vi "Audio Device Capture Example (G-Audio).vi"() -> ()   [LabVIEW 2020]
doc: "Simple example of audio device capture, saving the acquired data to a WAV file."
uses:
  Controls/Audio Device Config.ctl
  Controls/Audio Device Format.ctl
  Controls/Audio Device Info.ctl
  Controls/Audio Device Type.ctl
  Controls/Audio File Info.ctl
  Controls/WAV Codec Specific Info.ctl
  Controls/WAV Container Format.ctl
  Controls/WAV Data Format.ctl
  d37775a1-27ef-4781-ba3e-b38a0bb78134.vi
  7b5afa26-ffc7-4768-ab84-ffe08a27723a.vi
  Private/Result To Error.vi
  d37775a1-27ef-4781-ba3e-b38a0bb78134.vi/6b901882-6109-4f44-aca5-48e1525e5248.vi
  d37775a1-27ef-4781-ba3e-b38a0bb78134.vi/06c0137a-63d3-4e30-982f-115d83a1188c.vi
  Private/Get Configured Audio Device Info.vi
  7b5afa26-ffc7-4768-ab84-ffe08a27723a.vi/fba40667-3e21-44fa-934c-95909d78721c.vi
  d37775a1-27ef-4781-ba3e-b38a0bb78134.vi/6b901882-6109-4f44-aca5-48e1525e5248.vi/a9d2058a-38f9-4c88-a1a9-9bf864ebbde5.vi
  d37775a1-27ef-4781-ba3e-b38a0bb78134.vi/06c0137a-63d3-4e30-982f-115d83a1188c.vi/4b7b629c-2e91-4160-9820-a26af8f6e677.vi
  d37775a1-27ef-4781-ba3e-b38a0bb78134.vi/06c0137a-63d3-4e30-982f-115d83a1188c.vi/e7c4a249-ce38-42b4-8985-5fdb76b4ebfc.vi
  7b5afa26-ffc7-4768-ab84-ffe08a27723a.vi/fba40667-3e21-44fa-934c-95909d78721c.vi/4b7b629c-2e91-4160-9820-a26af8f6e677.vi
  7b5afa26-ffc7-4768-ab84-ffe08a27723a.vi/fba40667-3e21-44fa-934c-95909d78721c.vi/e7c4a249-ce38-42b4-8985-5fdb76b4ebfc.vi
  Audio Files/Polymorphic VIs/Open Audio File Write (WAV).vi
  <vilib>/Utility/Data Type/Get Numeric Information.vi
  <vilib>/Utility/error.llb/Error Cluster From Error Code.vi
  G-Audio.lvlib
panel:
  out "error out":errorcluster
  in  "Stop":bool
  out "Waveform":waveform(i16)[](graph)
  # "Instructions:\n1. Run the VI.\n2. Choose a WAV file location to save the captured audio data to.\n3. The VI will begin audio capture and display the data in the waveform graph.\n4. Press Stop to finish audio capture, and save the WAV fle.\n5. Listen to the recorded WAV with Audio Device Playback Example (G-Audio).vi."
  # "G"
  # "-Audio"
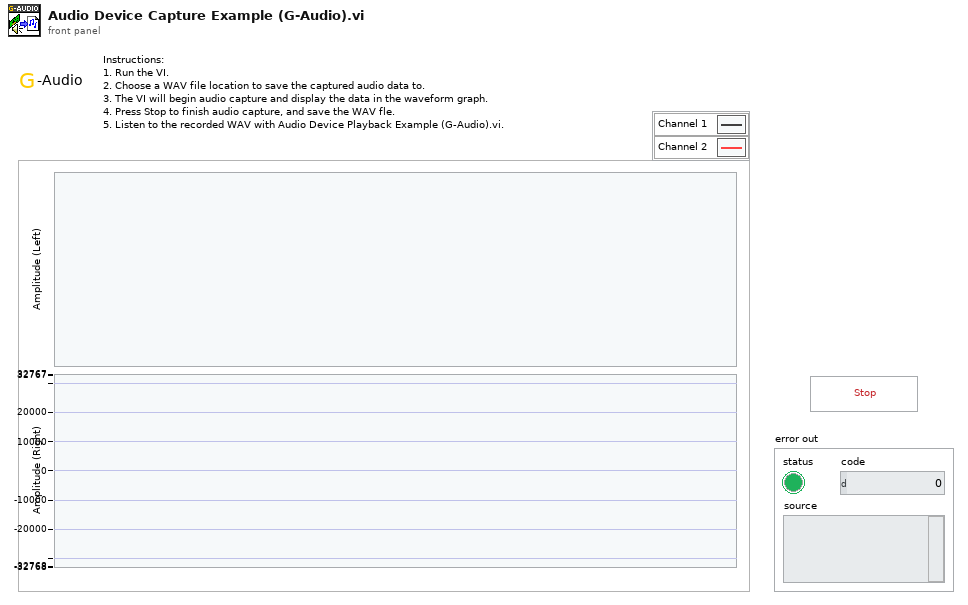
[diagram p1: front panel]
types:
  T1 = typedef "G-Audio.lvlib/WAV Codec Specific Info.ctl" = cluster{"Container Format":T2, "Data Format":T3}
  T2 = typedef "G-Audio.lvlib/WAV Container Format.ctl" = enum32{"RIFF", "Wave64"}
  T3 = typedef "G-Audio.lvlib/WAV Data Format.ctl" = u32
  T4 = typedef "G-Audio.lvlib/Audio File Info.ctl" = cluster{"Sample Rate (Hz)":u32, "Channels":u32, "Bit Depth":u32}
  T5 = typedef "G-Audio.lvlib/Audio Device Info.ctl" = cluster{"Name":string, "ID":u8[], "Device Type":T6}
  T6 = typedef "G-Audio.lvlib/Audio Device Type.ctl" = enum16{"(None)", "Playback", "Capture", "Duplex", "Loopback"}
  T7 = typedef "G-Audio.lvlib/Audio Device Config.ctl" = cluster{"Sample Rate (Hz)":u32, "Channels":u32, "Format":T8, "Exclusive Mode":bool}
  T8 = typedef "G-Audio.lvlib/Audio Device Format.ctl" = enum16{"Native", "U8", "I16", "I32", "SGL"}
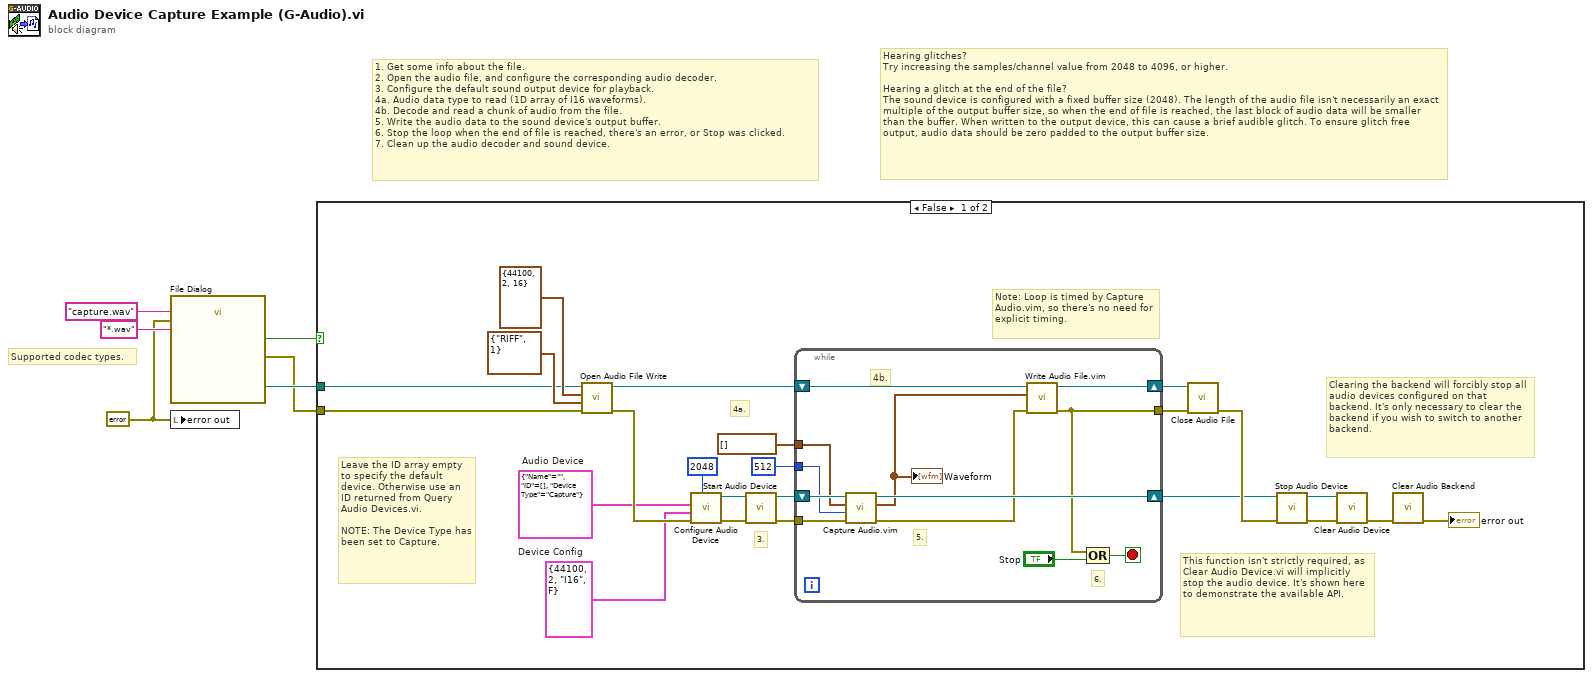
[diagram p0: block diagram]
diagram:
  w2 = errorcluster {"status"=FALSE, "code"=0, "source"=""} ("error out")
  # "Hearing glitches?\nTry increasing the samples/channel value from 2048 to 4096, or higher.\n\nHearing a glitch at the end of the file?\nThe sound device is configured with a fixed buffer size (2048). The length of the audio file isn't necessarily an exact multiple of the output buffer size, so when the end of file is reached, the last block of audio data will be smaller than the buffer. When written to the output device, this can cause a brief audible glitch. To ensure glitch free output, audio data should be zero padded to the output buffer size."
  # "1. Get some info about the file.\n2. Open the audio file, and configure the corresponding audio decoder.\n3. Configure the default sound output device for playback.\n4a. Audio data type to read (1D array of I16 waveforms).\n4b. Decode and read a chunk of audio from the file.\n5. Write the audio data to the sound device's output buffer.\n6. Stop the loop when the end of file is reached, there's an error, or Stop was clicked.\n7. Clean up the audio decoder and sound device."
  # "Supported codec types."
  n1 = call "File Dialog"("default name"="capture.wav", "error in"=w2, "pattern (all files)"="*.wav") -> ("selected path"=w5:path, "cancelled"=w4:bool, "error out"=w3:errorcluster)  [unwired: 9 in, 1 out]
  n2 = local write "error out"(w2) -> ()
  n3 = case shown="False" w4 {
    tunnel: w5 -> [w8 _]
    tunnel: w3 -> [w11 _]
    frame False {
      w12 = T5 {"Name"="", "ID"=[], "Device Type"=enum."Capture"}  # Audio Device
      w15 = T7 {"Sample Rate (Hz)"=44100, "Channels"=2, "Format"=enum."I16", "Exclusive Mode"=FALSE}  # Device Config
      # "Leave the ID array empty to specify the default device. Otherwise use an ID returned from Query Audio Devices.vi.\n\nNOTE: The Device Type has been set to Capture."
      # "This function isn't strictly required, as Clear Audio Device.vi will implicitly stop the audio device. It's shown here to demonstrate the available API."
      # "Clearing the backend will forcibly stop all audio devices configured on that backend. It's only necessary to clear the backend if you wish to switch to another backend."
      # "Note: Loop is timed by Capture Audio.vim, so there's no need for explicit timing."
      # "4a."
      # "3."
      n4 = call-poly "Open Audio File Write.vi"("error in (no error)"=w11, "Codec Specific Info"=T1 {"Container Format"=enum."RIFF", "Data Format"=1}, "Audio File Info"=T4 {"Sample Rate (Hz)"=44100, "Channels"=2, "Bit Depth"=16}, "Path"=w8) -> ("error out"=w19:errorcluster, "Audio File Refnum"=w21:refnum<file>)  [unwired: 6 in]
      n5 = call "Configure Audio Device.vi"("Buffer Size (4096)"=2048 ("number of samples/ch"), "error in (no error)"=w19, "Device Config"=w15, "Audio Device"=w12) -> ("error out"=w18:errorcluster, "Audio Device Refnum"=w17:refnum<file>)  [unwired: 6 in]
      n6 = call "Start Audio Device.vi"("error in (no error)"=w18, "Audio Device Refnum In"=w17) -> ("error out"=w23:errorcluster, "Audio Device Refnum Out"=w24:refnum<file>)  [unwired: 8 in]
      n7 = while {
        shift-right: [w39] -> w29
        shift-left: w21 -> [w41]
        shift-right: [w38] -> w13
        shift-left: w24 -> [w40]
        tunnel: w23 -> [w33]
        tunnel: [w31] -> w27
        tunnel: 512 ("number of samples/ch") -> [w35]
        tunnel: waveform(i16)[] [] -> [w34]
        stop <- w37 stop-if-true
        # "6."
        # "5."
        # "4b."
        n8 = call "Capture Audio.vim"("error in (no error)"=w33, "Samples To Read"=w35, "Data Format"=w34, "Audio Device Refnum In"=w40) -> ("error out"=w32:errorcluster, "Audio Data"=w30:waveform(i16)[], "Audio Device Refnum Out"=w38:refnum<file>)  [unwired: 5 in]
        "Waveform" <- w30
        n9 = call "Write Audio File.vim"("error in (no error)"=w32, "Audio Data"=w30, "Audio File Refnum In"=w41) -> ("error out"=w31:errorcluster, "Audio File Refnum Out"=w39:refnum<file>)  [unwired: 7 in]
        n10 = Compound Arithmetic op=OR(w31, "Stop") -> (w37:bool)
      }
      n11 = call "Close Audio File.vi"("error in (no error)"=w27, "Audio File Refnum In"=w29) -> ("error out"=w26:errorcluster)  [unwired: 9 in]
      n12 = call "Stop Audio Device.vi"("error in (no error)"=w26, "Audio Device Refnum In"=w13) -> ("error out"=w25:errorcluster, "Audio Device Refnum Out"=w28:refnum<file>)  [unwired: 8 in]
      n13 = call "Clear Audio Device.vi"("error in (no error)"=w25, "Audio Device Refnum In"=w28) -> ("error out"=w22:errorcluster)  [unwired: 9 in]
      n14 = call "Clear Audio Backend.vi"("error in (no error)"=w22) -> ("error out"=→"error out":errorcluster)  [unwired: 10 in]
    }
    frame True {
    }
  }
